vi "DecodeEnemyRobots.vi"(8 "error in":errorcluster, 9 "array":u8[](array[numeric]), 10 "Key":i32=5) -> (0 "error out":errorcluster, 1 "array w/ subset deleted out":u8[](array[numeric]), 3 "Enemy_Robots":T1(array[cluster]))   [LabVIEW 2017]
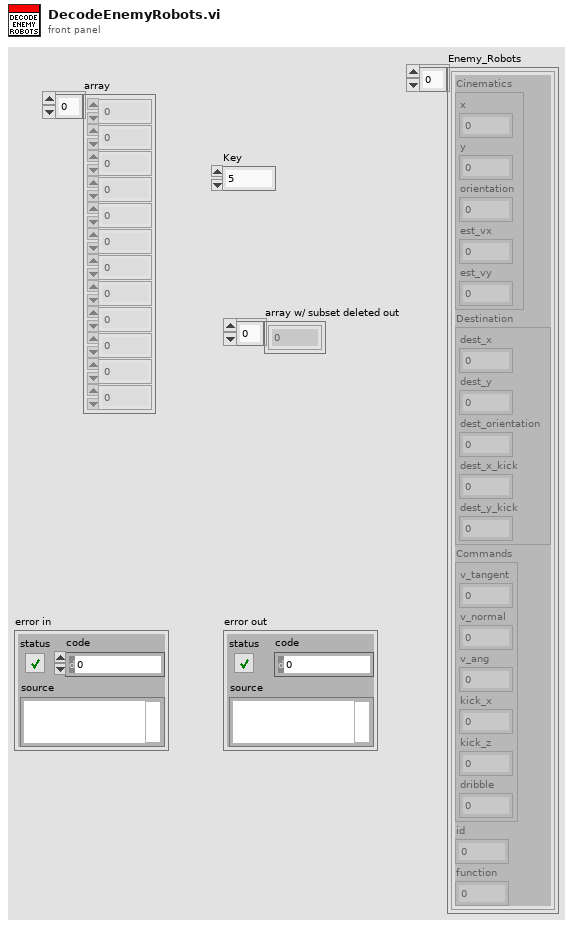
[diagram p1: front panel]
types:
  T1 = cluster{"Cinematics":cluster{"x":dbl, "y":dbl, "orientation":dbl, "est_vx":dbl, "est_vy":dbl}, "Destination":cluster{"dest_x":dbl, "dest_y":dbl, "dest_orientation":dbl, "dest_x_kick":dbl, "dest_y_kick":dbl}, "Commands":cluster{"v_tangent":dbl, "v_normal":dbl, "v_ang":dbl, "kick_x":dbl, "kick_z":dbl, "dribble":u32}, "id":u32, "function":u32}[]
  T2 = cluster{"Cinematics":cluster{"x":dbl, "y":dbl, "orientation":dbl, "est_vx":dbl, "est_vy":dbl}, "Destination":cluster{"dest_x":dbl, "dest_y":dbl, "dest_orientation":dbl, "dest_x_kick":dbl, "dest_y_kick":dbl}, "Commands":cluster{"v_tangent":dbl, "v_normal":dbl, "v_ang":dbl, "kick_x":dbl, "kick_z":dbl, "dribble":u32}, "id":u32, "function":u32}
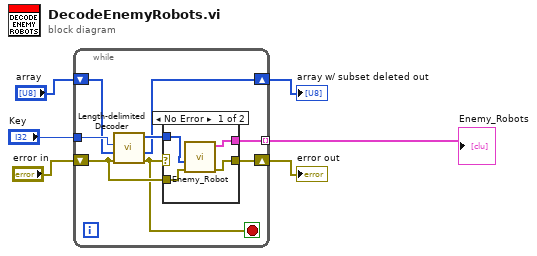
[diagram p0: block diagram]
diagram:
  n1 = while {
    tunnel: "Key" -> [w10]
    tunnel: [w8] -> w1 mode=indexing
    shift-right: [w12] -> w5
    shift-left: "error in" -> [w11]
    shift-right: [w13] -> w6
    shift-left: "array" -> [w9]
    stop <- w7 stop-if-true
    n2 = call "Length-delimited Decoder.vi"("error in (no error)"=w11, "Array"=w9, "Key"=w10) -> ("error out"=w7:errorcluster, "array w/ subset deleted"=w13:u8[], "Length-delimited"=w14:u8[])  [unwired: 5 in, 1 out]
    n3 = case shown="No Error" w7 {
      tunnel: [w16 w19] -> w12
      tunnel: w14 -> [w18 _]
      tunnel: w11 -> [w17 w19]
      tunnel: [w15 _] -> w8
      frame No Error {
        n4 = call "Enemy_Robot.vi"("error in"=w17, "Array"=w18) -> ("error out"=w16:errorcluster, "Enemy_Robots"=w15:T2)  [unwired: 7 in, 1 out]
      }
      frame Error {
      }
    }
  }
  "error out" <- w5
  "array w/ subset deleted out" <- w6
  "Enemy_Robots" <- w1
